vi "Elmo Read Status.vi"(11 "State Word":u16) -> (3 "Elmo State":T1)   [LabVIEW 2019]
uses:
  Elmo Status.ctl
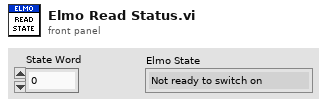
[diagram p1: front panel]
types:
  T1 = typedef "Elmo Status.ctl" = enum16{"Not ready to switch on", "Switch on disabled", "Ready to switch on", "Switch on", "Operation Enabled", "Quick stop active", "Fault reaction active", "Fault", "None"}
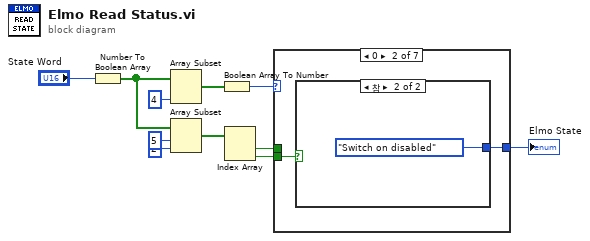
[diagram p0: block diagram]
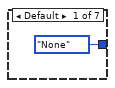
[diagram p2: hidden frame]
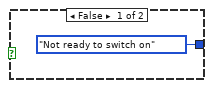
[diagram p3: hidden frame]
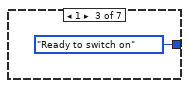
[diagram p4: hidden frame]
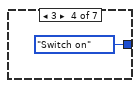
[diagram p5: hidden frame]
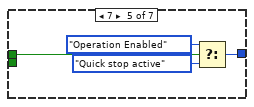
[diagram p6: hidden frame]
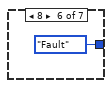
[diagram p7: hidden frame]
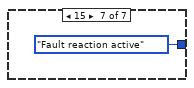
[diagram p8: hidden frame]
diagram:
  n1 = Number To Boolean Array(number="State Word") -> (Boolean array=w10:bool[])
  n2 = Array Subset(array=w10, length=4 ("길이")) -> (w6:bool[])  [unwired: 1 in]
  n3 = Array Subset(array=w10, index=5 ("인덱스"), length=2 ("길이")) -> (w4:bool[])
  n4 = Boolean Array To Number(Boolean array=w6) -> (number=w5:u32)
  n5 = Index Array(array=w4) -> (element #1=w1:bool, element #2=w3:bool)  [unwired: 2 in]
  n6 = case shown="0" w5 {
    tunnel: w3 -> [_ w14 _ _ _ _ _]
    tunnel: [Elmo_Status."None" ("Elmo State") w13 Elmo_Status."Ready to switch on" ("Elmo State") Elmo_Status."Switch on" ("Elmo State") w19 Elmo_Status."Fault" ("Elmo State") Elmo_Status."Fault reaction active" ("Elmo State")] -> w2
    tunnel: w1 -> [_ _ _ _ w22 _ _]
    frame Default {
    }
    frame 0 {
      n7 = case shown="참" w14 {
        tunnel: [Elmo_Status."Not ready to switch on" ("Elmo State") Elmo_Status."Switch on disabled" ("Elmo State")] -> w13
        frame False {
        }
        frame True {
        }
      }
    }
    frame 1 {
    }
    frame 3 {
    }
    frame 7 {
      n8 = Select(t=Elmo_Status."Operation Enabled" ("Elmo State"), s=w22, f=Elmo_Status."Quick stop active" ("Elmo State")) -> (s? t:f=w19:T1)
    }
    frame 8 {
    }
    frame 15 {
    }
  }
  "Elmo State" <- w2
